vi "Fit circle one.vi"(9 "Initial parameters":dbl[](array[numeric])=[188.484, 0.01, 2.4] format="%#_6p", 10 "Z":cdb[](array[numeric]), 11 "X":dbl[](array[numeric])) -> (1 "best fit parameters":dbl[](array[numeric]))   [LabVIEW 2016]
uses:
  <vilib>/gmath/NumericalOptimization/Nonlinear Curve Fit LM bound.vi
  <vilib>/gmath/NI_Gmath.lvlib
  <vilib>/Analysis/NI_AALPro.lvlib
panel:
  out "sqrt(x)":dbl
  out "Circle phase":dbl
  out "Circle plot":cluster{dbl[], dbl[]}[](graph)
  out "Phase in":cluster{"X":dbl[], dbl[]}(graph)
  out "Amplitude in":cluster{"X":dbl[], dbl[]}(graph)
  in  "Bounds":T1={"parameter minimum"=[1.0, 1.0, -6.3], "parameter maximum"=[10000000.0, 200.0, 10.0]} {"parameter minimum" format="%#_6p"}
  out "Weight":dbl[](graph)
  out "number of function calls":i32
  in  "termination":cluster{"max iteration":i32, "tolerance":dbl}={"max iteration"=200, "tolerance"=1e-08}
  out "Fit":cluster{"X":dbl[], "best nonlinear fit":dbl[]}[](graph)
  # "F0\nG\nA\nP\nX\nY"
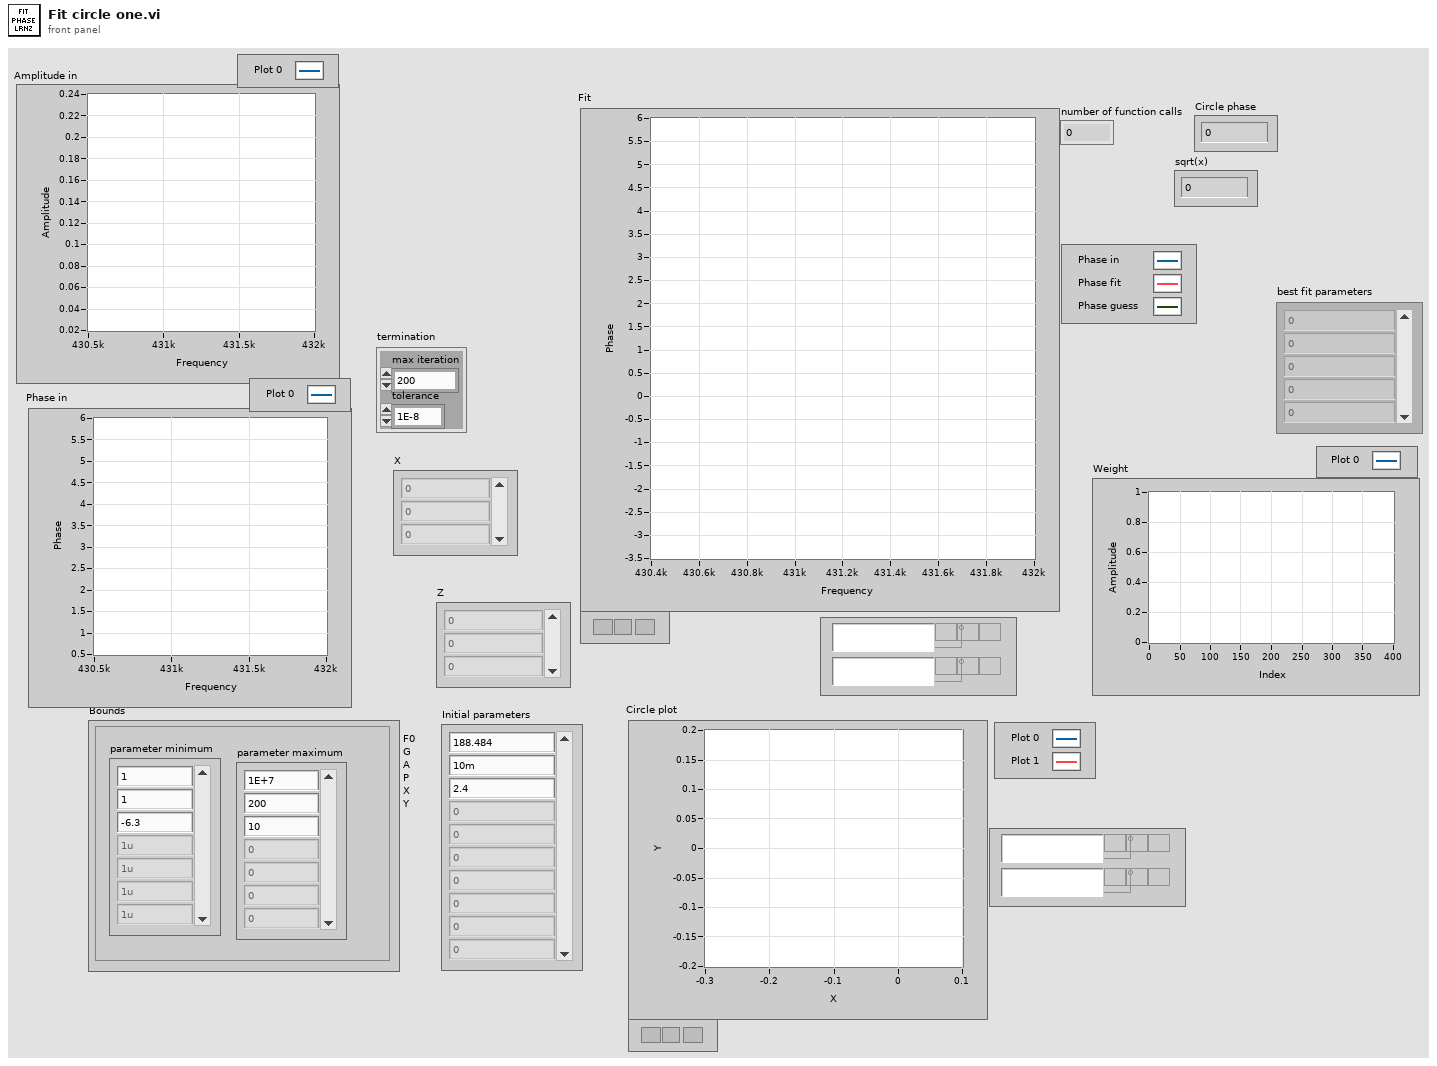
[diagram p1: front panel]
types:
  T1 = cluster{"parameter minimum":dbl[], "parameter maximum":dbl[]}
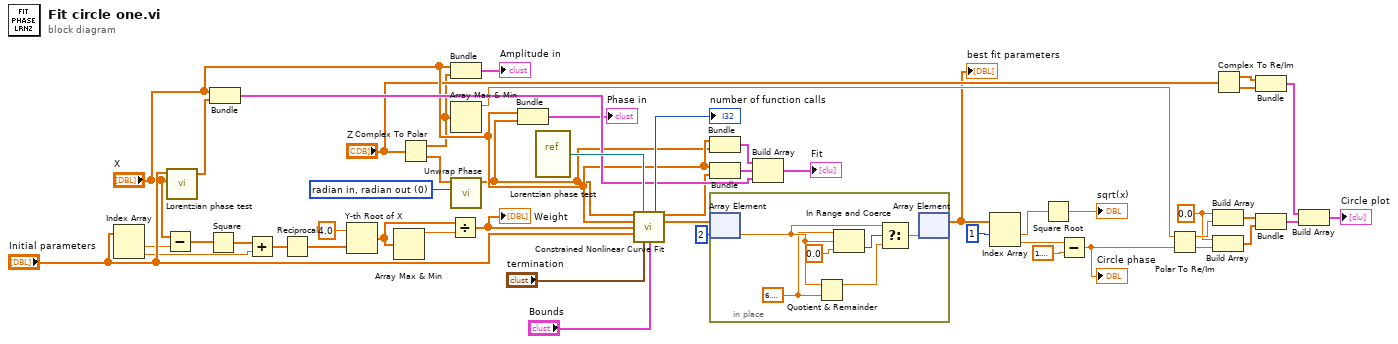
[diagram p0: block diagram]
diagram:
  w11 = 0 items=["radian in, radian out", "radian in, degree out", "degree in, degree out", "degree in, radian out"] ("phase unit")
  w22 = 0.0 ("element")
  n1 = Index Array(array="Initial parameters") -> (element #1=w40:dbl, element #2=w37:dbl)  [unwired: 2 in]
  n2 = Subtract(x="X", y=w40) -> (x-y=w39:dbl[])
  n3 = call "Lorentzian phase test.vi"("X"="X", "a"="Initial parameters") -> ("f(X,a)"=w42:dbl[])  [unwired: 2 in, 2 out]
  n4 = Square(x=w39) -> (x^2=w38:dbl[])
  n5 = Bundle("X"="X", "f(X,a)"=w42) -> (w45:cluster{"X":dbl[], "f(X,a)":dbl[]})  [unwired: 1 in]
  n6 = Add(x=w38, y=w37) -> (x+y=w36:dbl[])
  n7 = Reciprocal(x=w36) -> (1/x=w6:dbl[])
  n8 = Y-th Root of X(1:w6, 2:4.0) -> (0:w4:dbl[])
  n9 = Array Max & Min(array=w4) -> (max value=w35:dbl)  [unwired: 3 out]
  n10 = Complex To Polar(r * e^(i*theta)="Z") -> (r=w25:dbl[], theta=w10:dbl[])
  n11 = Divide(x=w4, y=w35) -> (x/y=w8:dbl[])
  "Weight" <- w8
  n12 = Bundle("X"="X", w25) -> (→"Amplitude in":cluster{"X":dbl[], dbl[]})  [unwired: 1 in]
  n13 = Array Max & Min(array=w25) -> (max value=w24:dbl)  [unwired: 3 out]
  n14 = call <vilib>:"Unwrap Phase.vi"("phase unit"=w11, "Phase"=w10) -> ("Unwrapped Phase"=w9:dbl[])  [unwired: 8 in, 1 out]
  n15 = Bundle("X"="X", "Unwrapped Phase"=w9) -> (→"Phase in":cluster{"X":dbl[], "Unwrapped Phase":dbl[]})  [unwired: 1 in]
  n16 = vi-ref "Lorentzian phase test.vi"() -> (w49:refnum<vi>)
  n17 = call-poly <vilib>:"Constrained Nonlinear Curve Fit.vi"("Y"=w9, "f(x,a)"=w49, "X"="X", "Weight"=w8, "initial parameters"="Initial parameters", "termination"="termination", "parameter bounds"="Bounds") -> ("number of function calls"=→"number of function calls":i32, "best nonlinear fit"=w30:dbl[], "best fit parameters"=w3:dbl[])  [unwired: 3 in, 3 out]
  n18 = Bundle("X"="X", "Unwrapped Phase"=w9) -> (w44:cluster{"X":dbl[], "Unwrapped Phase":dbl[]})  [unwired: 1 in]
  n19 = Bundle("X"="X", "best nonlinear fit"=w30) -> (w43:cluster{"X":dbl[], "best nonlinear fit":dbl[]})  [unwired: 1 in]
  n20 = in-place {
    w52 = 6.283185307179586
    n21 = in-place-array #1(w3, 2) -> (w53:dbl)
    n22 = Quotient & Remainder(x=w53, y=w52) -> (x-y*floor(x/y)=w51:dbl)  [unwired: 1 out]
    n23 = In Range and Coerce(upper limit=w52, x=w53, lower limit=0.0) -> (In Range?=w54:bool)  [unwired: 1 out]
    n24 = Select(t=w53, s=w54, f=w51) -> (s? t:f=w50:dbl)
    n25 = in-place-array #1(w50) -> (w2:dbl[])  [unwired: 1 out]
  }
  "best fit parameters" <- w2
  n26 = Build Array(w44, w43, w45) -> (→"Fit":cluster{"X":dbl[], "f(X,a)":dbl[]}[])
  n27 = Index Array(array=w2, index #1=1 ("index")) -> (element #1=w13:dbl, element #2=w14:dbl)  [unwired: 1 in]
  n28 = Square Root(x=w13) -> (sqrt(x)=→"sqrt(x)":dbl)
  n29 = Subtract(x=w14, y=1.5707963267948966) -> (x-y=w7:dbl)
  "Circle phase" <- w7
  n30 = Polar To Re/Im(2:w7, 3:w24) -> (0:w21:dbl, 1:w23:dbl)
  n31 = Build Array(w22, w23) -> (w20:dbl[])
  n32 = Build Array(w22, w21) -> (w19:dbl[])
  n33 = Complex To Re/Im(x + iy="Z") -> (x=w28:dbl[], y=w27:dbl[])
  n34 = Bundle(w28, w27) -> (w26:cluster{dbl[], dbl[]})  [unwired: 1 in]
  n35 = Bundle(w20, w19) -> (w17:cluster{dbl[], dbl[]})  [unwired: 1 in]
  n36 = Build Array(w26, w17) -> (→"Circle plot":cluster{dbl[], dbl[]}[])
